vi "Get SMO HELP.vi"(8 "error in (no error)":errorcluster, 10 "Command":string, 11 "Instrument.Amplifier in":refnum<class "Instrument.Amplifier.lvclass">) -> (0 "error out":errorcluster, 2 "help cluster":T1, 3 "Instrument.Amplifier out":refnum<class "Instrument.Amplifier.lvclass">)   [LabVIEW 2019, in "Instrument.Amplifier.lvclass"]
uses:
  Instrument.Amplifier.lvclass
  subsystems/Help/typedefs/Help--cluster.ctl
  Amplifier.Commands--Enum.ctl
  Instrument/Instrument.lvclass
  subsystems/Help/Help.lvclass
  Instrument/Typedefs/Instrument.Commands--Enum.ctl
  Instrument/Typedefs/Instrument.IDN--cluster.ctl
  <vilib>/ciozi137/JSON-Schema/JSON-Schema.lvlib
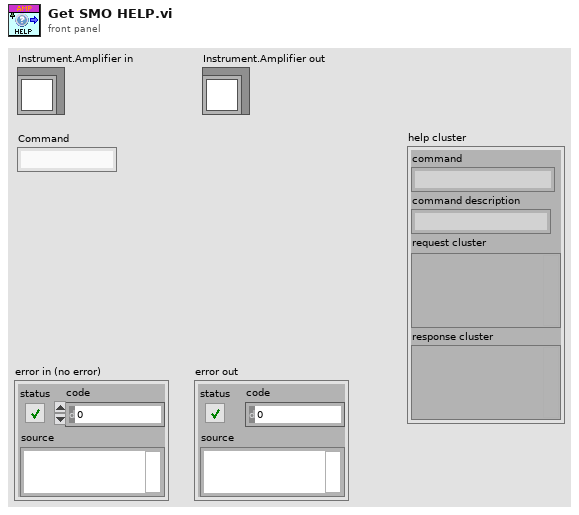
[diagram p1: front panel]
types:
  T1 = typedef "Instrument.lvlib/Help.lvclass/Help--cluster.ctl" = cluster{"command":string, "command description":string, "request cluster":variant, "response cluster":variant}
  T2 = typedef "Instrument.lvlib/Instrument.lvclass/Instrument.Commands--Enum.ctl" = enum16{"ACK", "HELP", "IDN", "getAll", "getAllData"}
  T3 = typedef "Instrument.lvlib/Instrument.lvclass/Instrument.IDN--cluster.ctl" = cluster{"vendor":string, "model":string, "serial":string, "firmware":string}
  T4 = typedef "Instrument.Amplifier.lvclass/Amplifier.Commands--Enum.ctl" = enum16{"getChannel", "getAllChannels", "setChannel", "setAllChannels"}
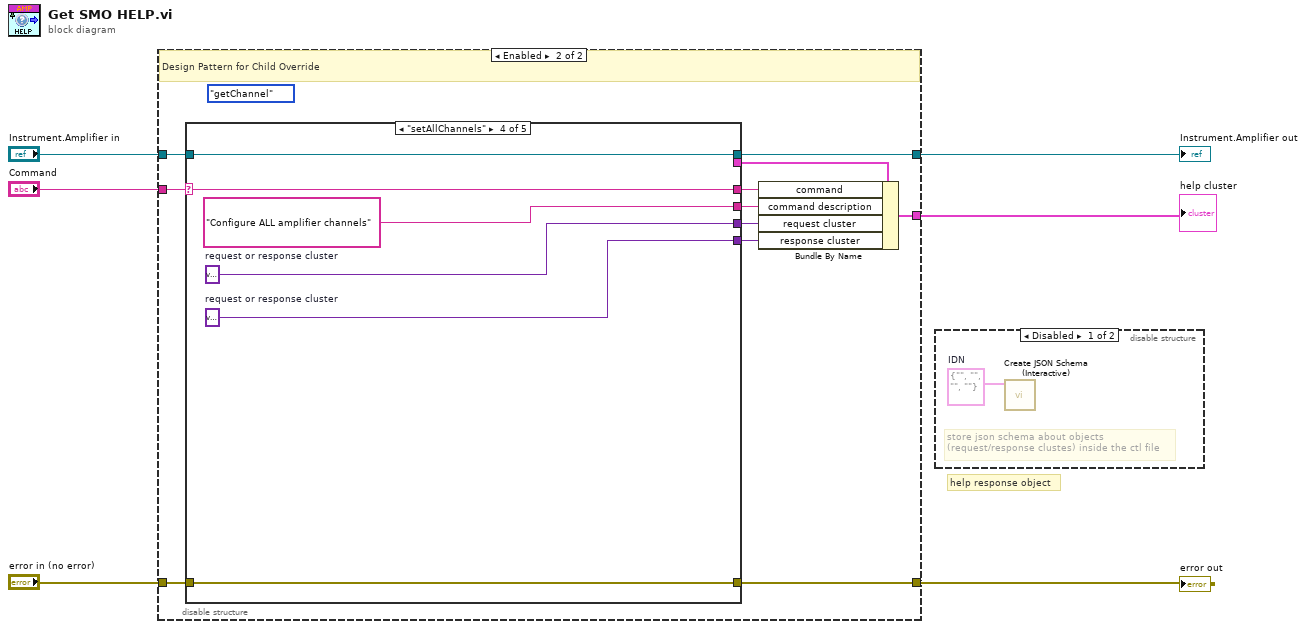
[diagram p0: block diagram]
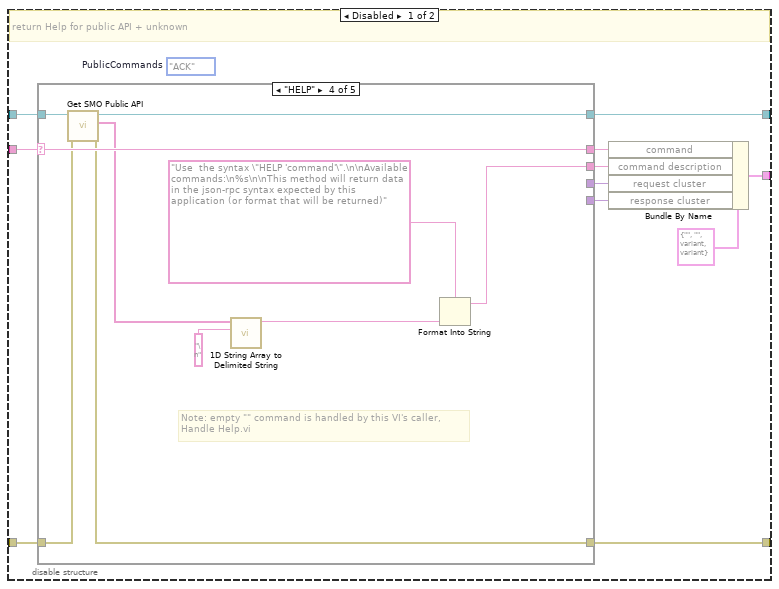
[diagram p3: hidden frame]
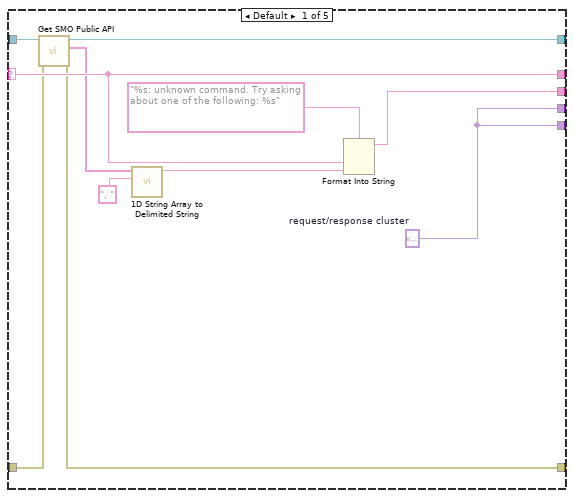
[diagram p4: hidden frame]
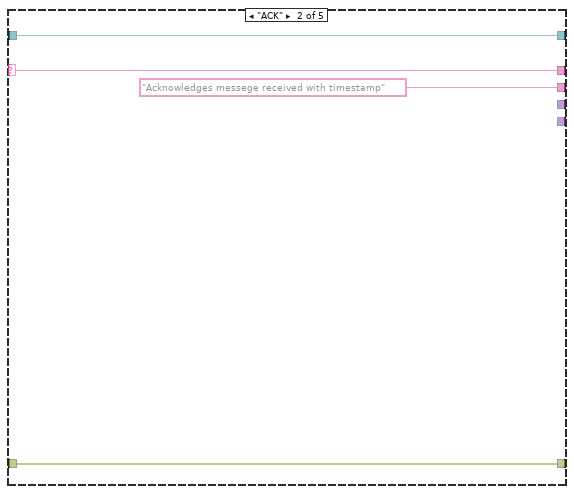
[diagram p5: hidden frame]
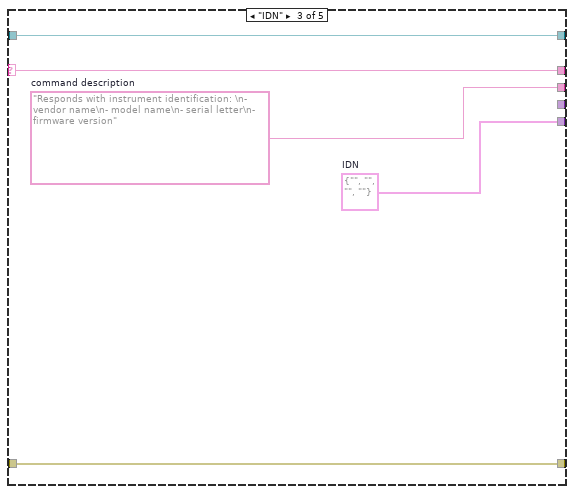
[diagram p6: hidden frame]
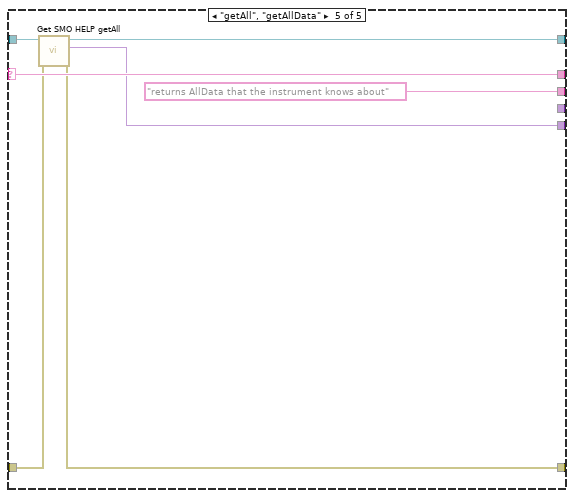
[diagram p7: hidden frame]
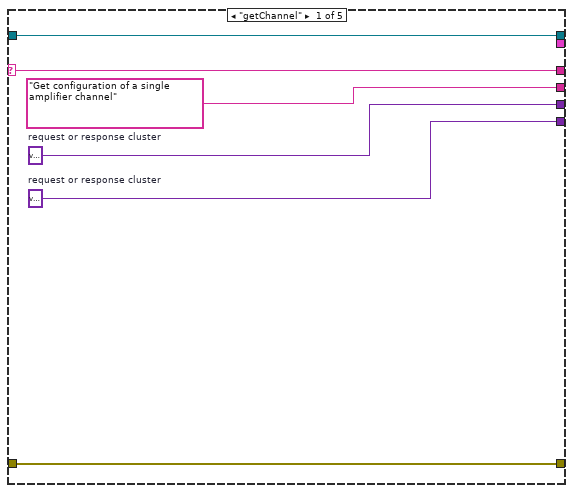
[diagram p8: hidden frame]
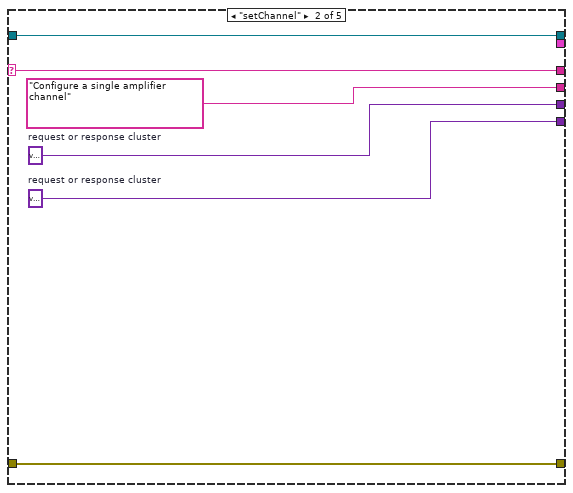
[diagram p9: hidden frame]
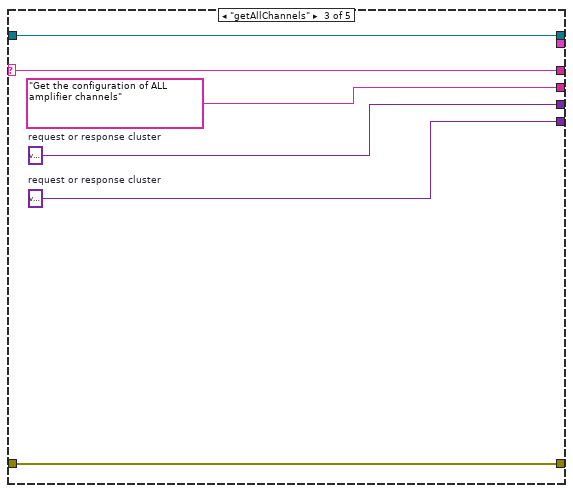
[diagram p10: hidden frame]
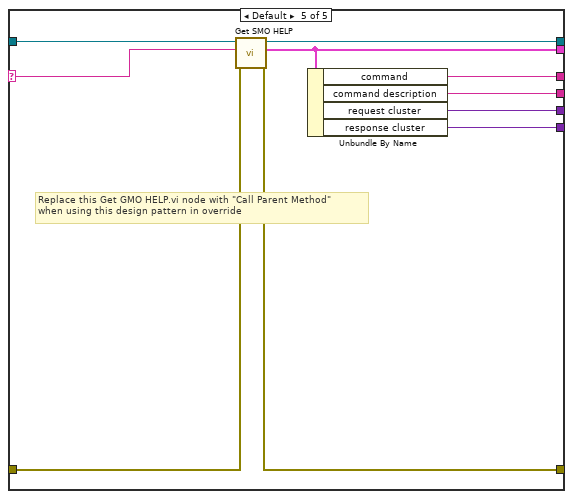
[diagram p11: hidden frame]
diagram:
  # "help response object"
  n1 = disable-structure shown="Enabled" {
    disable-tunnel: [w17 w56] -> w4
    disable-tunnel: "Instrument.Amplifier in" -> [w16 w57]
    disable-tunnel: "error in (no error)" -> [w15 w63]
    disable-tunnel: [w11 w65] -> w6
    disable-tunnel: [w8 w64] -> w5
    disable-tunnel: "Command" -> [w7 w62]
    frame Disabled {
      (unwired) Instrument.Commands--Enum."ACK"  # PublicCommands
      # "return Help for public API + unknown"
      n2 = case shown="\"HELP\"" w7 {
        selector: w7 -> [w24 w30 w36 w44 w53]
        tunnel: w15 -> [w21 w32 w34 w41 w52]
        tunnel: [w22 w32 w34 w42 w51] -> w11
        tunnel: [w26 "Acknowledges messege received with timestamp" w37 w38 "returns AllData that the instrument knows about"] -> w13
        tunnel: [w19 _ _ _ _] -> w12
        tunnel: [w19 _ w33 _ w48] -> w10
        tunnel: [w24 w30 w36 w44 w53] -> w14
        tunnel: w16 -> [w23 w29 w35 w43 w49]
        tunnel: [w20 w29 w35 w40 w50] -> w17
        frame Default {
          w19 = variant  # request/response cluster
          n3 = call-dynamic "Get SMO Public API.vi"("error in (no error)"=w21, "Instrument.Amplifier in"=w23) -> ("error out"=w22:errorcluster, "commands"=w18:string[], "Instrument.Amplifier out"=w20:refnum<class "Instrument.Amplifier.lvclass">)  [unwired: 7 in]
          n4 = call <vilib>:"1D String Array to Delimited String.vi"("delimiter"=", ", "string array"=w18) -> ("delimited string"=w27:string)  [unwired: 9 in]
          n5 = Format Into String(format string="%s: unknown command. Try asking about one of the following: %s", w24, w27) -> (resulting string=w26:string)  [unwired: 2 in, 1 out]
        }
        frame "ACK" {
        }
        frame "IDN" {
          w33 = T3 {"vendor"="", "model"="", "serial"="", "firmware"=""}  # IDN
          w37 = "Responds with instrument identification: \n- vendor name\n- model name\n- serial letter\n- firmware version"  # command description
        }
        frame "HELP" {
          # "Note: empty \"\" command is handled by this VI's caller,\nHandle Help.vi"
          n6 = call-dynamic "Get SMO Public API.vi"("error in (no error)"=w41, "Instrument.Amplifier in"=w43) -> ("error out"=w42:errorcluster, "commands"=w39:string[], "Instrument.Amplifier out"=w40:refnum<class "Instrument.Amplifier.lvclass">)  [unwired: 7 in]
          n7 = call <vilib>:"1D String Array to Delimited String.vi"("delimiter"="\n", "string array"=w39) -> ("delimited string"=w47:string)  [unwired: 9 in]
          n8 = Format Into String(format string="Use  the syntax \"HELP 'command'\".\n\nAvailable commands:\n%s\n\nThis method will return data in the json-rpc syntax expected by this application (or format that will be returned)", w47) -> (resulting string=w38:string)  [unwired: 2 in, 1 out]
        }
        frame "getAll", "getAllData" {
          n9 = call-dynamic "Get SMO HELP getAll.vi"("error in (no error)"=w52, "Instrument in"=w49) -> ("error out"=w51:errorcluster, "response cluster"=w48:variant, "Instrument out"=w50:refnum<class "Instrument.Amplifier.lvclass">)  [unwired: 7 in]
        }
      }
      n10 = Bundle By Name(cluster=T1 {"command"="", "command description"="", "request cluster"=variant, "response cluster"=variant} ("Help"), "command"=w14, "command description"=w13, "request cluster"=w12, "response cluster"=w10) -> (w8:T1)
    }
    frame Enabled {
      (unwired) Amplifier.Commands--Enum."getChannel" ("Commands")
      # "Design Pattern for Child Override"
      n11 = case shown="\"setAllChannels\"" w62 {
        selector: w62 -> [w71 w77 w83 w89 w98]
        tunnel: [w71 w77 w83 w89 w93] -> w61
        tunnel: w63 -> [w70 w76 w82 w88 w91]
        tunnel: [w70 w76 w82 w88 w90] -> w65
        tunnel: ["Get configuration of a single amplifier channel" "Configure a single amplifier channel" "Get the configuration of ALL amplifier channels" "Configure ALL amplifier channels" w94] -> w60
        tunnel: [w68 w74 w80 w86 w95] -> w59
        tunnel: [w67 w73 w79 w85 w96] -> w58
        tunnel: w57 -> [w66 w72 w78 w84 w99]
        tunnel: [w66 w72 w78 w84 w97] -> w56
        tunnel: [_ _ _ _ w92] -> w55
        frame "getChannel" {
          w68 = variant  # request or response cluster
          w67 = variant  # request or response cluster
        }
        frame "setChannel" {
          w74 = variant  # request or response cluster
          w73 = variant  # request or response cluster
        }
        frame "getAllChannels" {
          w80 = variant  # request or response cluster
          w79 = variant  # request or response cluster
        }
        frame "setAllChannels" {
          w86 = variant  # request or response cluster
          w85 = variant  # request or response cluster
        }
        frame Default {
          # "Replace this Get GMO HELP.vi node with \"Call Parent Method\"\nwhen using this design pattern in override"
          n12 = call-parent "Get SMO HELP.vi"("error in (no error)"=w91, "Command"=w98, "Instrument in"=w99) -> ("error out"=w90:errorcluster, "help cluster"=w92:T1, "Instrument out"=w97:refnum<class "Instrument.Amplifier.lvclass">)  [unwired: 6 in]
          n13 = Unbundle By Name(w92) -> ("command"=w93:string, "command description"=w94:string, "request cluster"=w95:variant, "response cluster"=w96:variant)
        }
      }
      n14 = Bundle By Name(cluster=w55, "command"=w61, "command description"=w60, "request cluster"=w59, "response cluster"=w58) -> (w64:T1)
    }
  }
  "Instrument.Amplifier out" <- w4
  "help cluster" <- w5
  "error out" <- w6
  n15 = disable-structure shown="Disabled" {
    frame Disabled {
      w100 = T3 {"vendor"="", "model"="", "serial"="", "firmware"=""}  # IDN
      # "store json schema about objects\n(request/response clustes) inside the ctl file"
      n16 = call <vilib>:"Create JSON Schema (Interactive).vi"(10:w100) -> ()  [unwired: 9 in, 2 out]
    }
    frame Enabled {
    }
  }
